vi "zern.vi"(6 "A":dbl, 7 "R":dbl, 9 "m":i32, 10 "n":i32, 11 "field":T1) -> (3 "field out":T1)   [LabVIEW 2012, in "LightPipes.lvlib"]
doc: "__declspec(dllexport) void zern(FIELD *field, int n, int m, double R, double A);"
uses:
  LightPipes.lvlib
  Lightpipes.dll
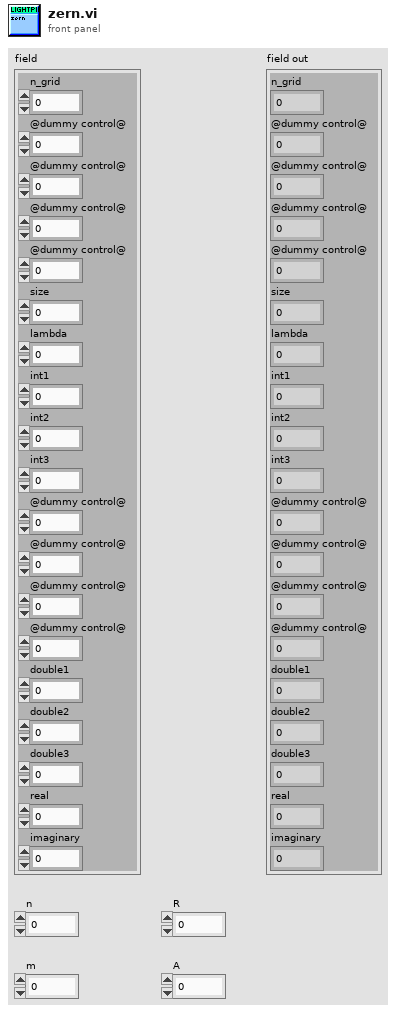
[diagram p1: front panel]
types:
  T1 = cluster{"n_grid":i32, "@dummy control@":i8, "@dummy control@":i8, "@dummy control@":i8, "@dummy control@":i8, "size":dbl, "lambda":dbl, "int1":i32, "int2":i32, "int3":i32, "@dummy control@":i8, "@dummy control@":i8, "@dummy control@":i8, "@dummy control@":i8, "double1":dbl, "double2":dbl, "double3":dbl, "real":u32, "imaginary":u32}
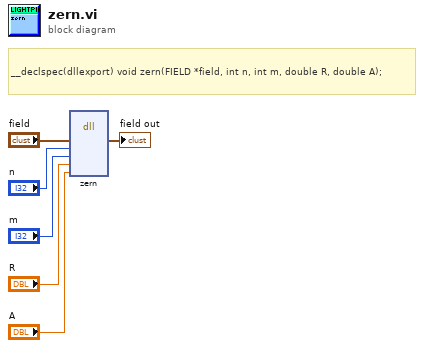
[diagram p0: block diagram]
diagram:
  # "__declspec(dllexport) void zern(FIELD *field, int n, int m, double R, double A);"
  n1 = dll-call lib="C:/Users/Tri/Documents/Lightpipes/LabView/Lightpipes.*" fn="zern"("field"="field", "n"="n", "m"="m", "R"="R", "A"="A") -> ("field"=→"field out":T1)  [unwired: 8 in, 2 out]
